vi "Reserve.vi"(0 "SLSC Remote in":refnum<class "SLSC Remote.lvclass">, 11 "error in (no error)":errorcluster) -> (4 "SLSC Remote out":refnum<class "SLSC Remote.lvclass">, 15 "error out":errorcluster)   [LabVIEW 2015, in "SLSC Remote.lvclass"]
uses:
  SLSC Remote.lvclass
  <vilib>/NI/i3 JSON/JSON Generation/Create Value Files/Create Value - Object.vi
  <vilib>/NI/i3 JSON/JSON Generation/Add Object Parameter Files/Add Object Parameter - String.vi
  <vilib>/NI/NI JSONRPC Server Framework/Classes/Server/Format Client Request (Auto-Increment).vi
  <vilib>/httpClient/POSTBuffer.vi
  <vilib>/NI/NI JSONRPC Server Framework/Classes/Server/JSONRPC Server.lvclass
  <vilib>/NI/i3 JSON/i3-json.lvlib
  <vilib>/httpClient/LabVIEWHTTPClient.lvlib
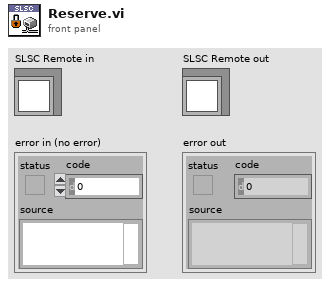
[diagram p1: front panel]
types:
  T1 = typedef "LabVIEWHTTPClient.lvlib/ClientHandle.ctl" = refnum<k1>
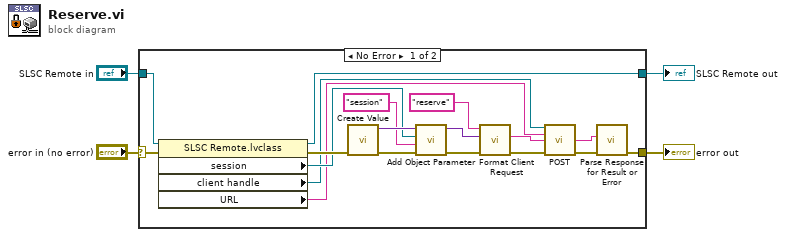
[diagram p0: block diagram]
diagram:
  n1 = case shown="No Error" "error in (no error)" {
    selector: "error in (no error)" -> [w19 w23]
    tunnel: "SLSC Remote in" -> [w21 w24]
    tunnel: [w20 w24] -> w3
    tunnel: [w5 w23] -> w1
    frame No Error {
      n2 = property class="SLSC Remote.lvclass"(reference=w21, error in=w19) -> (reference out=w20:refnum<class "SLSC Remote.lvclass">, error out=w18:errorcluster, "session"=w14:refnum<k21>, "client handle"=w10:T1, "URL"=w9:string)
      n3 = call-poly <vilib>:"Create Value.vi"("error in (no error)"=w18) -> ("error out"=w17:errorcluster, "JSON Tree"=w22:variant)  [unwired: 9 in]
      n4 = call-poly <vilib>:"Add Object Parameter.vi"("error in (no error)"=w17, "Name"="session", "String"=w14, "JSON Tree in (JSON Object)"=w22) -> ("error out"=w11:errorcluster, "JSON Tree out (JSON Object)"=w12:variant)  [unwired: 6 in]
      n5 = call-poly <vilib>:"Format Client Request.vi"("error in (no error)"=w11, "params"=w12, "method"="reserve") -> ("error out"=w8:errorcluster, "Request String"=w15:string)  [unwired: 7 in]
      n6 = call-poly <vilib>:"POST.vi"("client handle"=w10, "url"=w9, "buffer"=w15, "error in (no error)"=w8) -> ("body"=w7:string, "error out"=w6:errorcluster)  [unwired: 8 in, 2 out]
      n7 = call <vilib>:"Parse Response for Result or Error.vi"("error in"=w6, "Response String In"=w7) -> ("error out"=w5:errorcluster)  [unwired: 8 in, 1 out]
    }
    frame Error {
    }
  }
  "error out" <- w1
  "SLSC Remote out" <- w3
